vi "Pneumatic Sucker Suck.vi"(8 "error in":errorcluster, 10 "suck sec":dbl=0.8 format="%#_13g") -> (0 "error out":errorcluster)   [LabVIEW 2019]
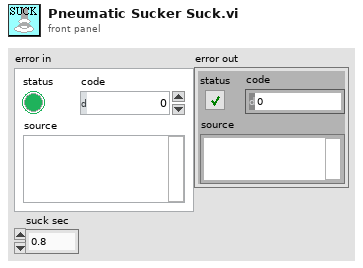
[diagram p1: front panel]
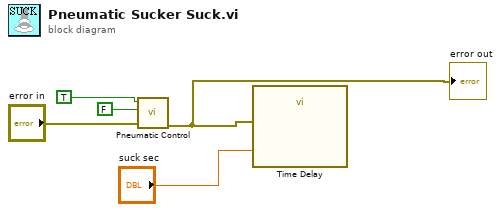
[diagram p0: block diagram]
diagram:
  n1 = call "Pneumatic Control.vi"("error in"="error in", "DIR"=FALSE, "ENA"=TRUE) -> ("error out"=w1:errorcluster)  [unwired: 8 in]
  "error out" <- w1
  n2 = call "Time Delay"("error in (no error)"=w1, "Delay Time (s)"="suck sec") -> ()  [unwired: 9 in, 1 out]
